vi "Test DSCConnection.vi"() -> ()   [LabVIEW 2014]
doc: "Create/Open/Write Shared Variable. Create Process if not existing."
uses:
  CSPP_Core/Classes/CS++BaseClasses/Factory/CS++Factory.lvclass
  CSPP_Core/Libraries/Base/FGV Action.ctl
  CSPP_Core/Classes/CS++ProcessVariables/ProcessVariable/PV.lvclass
  Actors/CS++DSCManager/CS++DSCManager.lvclass
  CSPP_Core/Classes/CS++BaseClasses/Factory/CS++Factory.lvclass/CS++Factory.ctl
  CSPP_Core/Classes/CS++ProcessVariables/ProcessVariable/PV.lvclass/PV.ctl
  CSPP_Core/Classes/CS++ProcessVariables/ProcessVariable/Write PV URL.vi
  CSPP_Core/Classes/CS++ProcessVariables/ProcessVariable/Write Type Descriptor.vi
  CSPP_Core/Classes/CS++ProcessVariables/ProcessVariable/Write Data.vi
  CSPP_Core/Classes/CS++ProcessVariables/ProcessVariable/Read Data.vi
  CSPP_Core/Classes/CS++ProcessVariables/CS++ProcessVariables.lvlib
  CSPP_Core/Libraries/Base/CS++Base.lvlib
  CSPP_Core/Classes/CS++ProcessVariables/PVConnection/PVConnection.lvclass
panel:
  out "data":dbl
  in  "SV-Lib":path=path "C:/tmp/myProcess.lvlib"
  out "Error Out":errorcluster
  in  "Value":dbl=40.0
  out "Success":bool=TRUE
  in  "Access (R/W allowed)":T1
  in  "PV URL":string="ni.var.psp://localhost/myProcess/myDouble"
  in  "Ini-file":path=path "C:/User/Brand/LVP/CSPP-Dev/CS++Dev.ini"
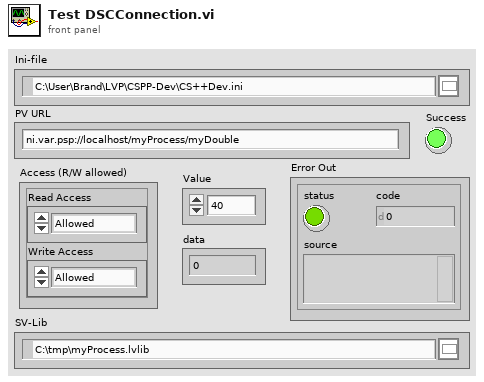
[diagram p1: front panel]
types:
  T1 = cluster{"Read Access":enum8{"Allowed", "Required", "None"}, "Write Access":enum8{"Allowed", "Required", "None"}}
  T2 = typedef "CS++Base.lvlib/FGV Action.ctl" = enum16{"add", "replace", "read", "remove", "reset", "get attributes"}
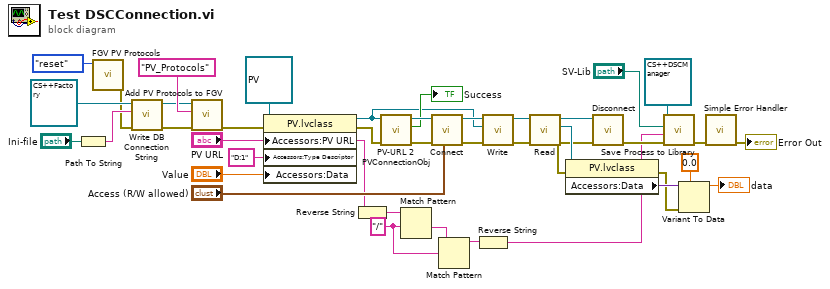
[diagram p0: block diagram]
diagram:
  w12 = "/" ("regular expression")
  n1 = Path To String(path="Ini-file") -> (string=w36:string)
  n2 = call "FGV PV Protocols.vi"("Action (read)"=FGV_Action."reset") -> ("Error Out"=w33:errorcluster)  [unwired: 6 in, 4 out]
  n3 = call "Write DB Connection String.vi"("error in (no error)"=w33, "DB Connection String"=w36, "CS++Factory in"=refnum<class "CS++Factory.lvclass"> refnum ("CS++Factory")) -> ("error out"=w35:errorcluster, "CS++Factory out"=w38:refnum<class "CS++Factory.lvclass">)  [unwired: 7 in]
  n4 = call "Add PV Protocols to FGV.vi"("Error In"=w35, "PV Protocol Section"="PV_Protocols" ("string"), "CS++Factory"=w38) -> ("Error Out"=w31:errorcluster)  [unwired: 8 in]
  n5 = property class="PV.lvclass"(reference=refnum<class "PV.lvclass"> refnum ("CS++ProcessVariables.lvlib:PV.lvclass"), error in=w31, "Accessors:PV URL"="PV URL", "Accessors:Type Descriptor"="D:1" ("Type Descriptor"), "Accessors:Data"="Value") -> (reference out=w22:refnum<class "PV.lvclass">, error out=w29:errorcluster)
  n6 = Reverse String(1:"PV URL") -> (0:w15:string)
  n7 = call "PV-URL 2 PVConnectionObj.vi"("Error In"=w29, "PV"=w22) -> ("Error Out"=w27:errorcluster, "Success"=→"Success":bool, "PVConnection"=w28:refnum<class "PVConnection.lvclass">)  [unwired: 7 in]
  n8 = Match Pattern(string=w15, regular expression=w12) -> (after substring=w13:string)  [unwired: 1 in, 3 out]
  n9 = call "Connect.vi"("Access (R/W allowed)"="Access (R/W allowed)", "error in (no error)"=w27, "PVConnection in"=w28) -> ("error out"=w24:errorcluster, "PVConnection out"=w25:refnum<class "PVConnection.lvclass">)  [unwired: 7 in]
  n10 = Match Pattern(string=w13, regular expression=w12) -> (before substring=w11:string)  [unwired: 1 in, 3 out]
  n11 = Reverse String(1:w11) -> (0:w10:string)
  n12 = call "Write.vi"("error in (no error)"=w24, "PV"=w22, "PVConnection in"=w25) -> ("error out"=w7:errorcluster, "PVConnection out"=w9:refnum<class "PVConnection.lvclass">)  [unwired: 7 in]
  n13 = call "Read.vi"("error in (no error)"=w7, "PVConnection in"=w9) -> ("error out"=w5:errorcluster, "PV"=w6:refnum<class "PV.lvclass">, "PVConnection out"=w8:refnum<class "PVConnection.lvclass">)  [unwired: 6 in, 1 out]
  n14 = property class="PV.lvclass"(reference=w6, error in=w5) -> (error out=w3:errorcluster, "Accessors:Data"=w4:variant)  [unwired: 1 out]
  n15 = call "Disconnect.vi"("error in (no error)"=w5, "PVConnection in"=w8) -> ("error out"=w17:errorcluster)  [unwired: 8 in, 1 out]
  n16 = call "Save Process to Library.vi"("Error In"=w17, "Process"=w10, "Library Path"="SV-Lib", "CS++DSCManager in"=refnum<class "CS++DSCManager.lvclass"> refnum ("CS++DSCManager.lvlib:CS++DSCManager.lvclass")) -> ("Error Out"=w16:errorcluster)  [unwired: 5 in, 2 out]
  n17 = Variant To Data(error in=w3, type=0.0, Variant=w4) -> (data=→"data":dbl)  [unwired: 1 out]
  n18 = call <vilib>:"Simple Error Handler.vi"("error in (no error)"=w16) -> ("error out"=→"Error Out":errorcluster)  [unwired: 4 in, 4 out]
